vi "Flip Matrix.vi"(8 "Error In":errorcluster, 11 "Frame In":u32[][](array[numeric])) -> (0 "Error Out":errorcluster, 3 "Frame Out":u32[][](array[numeric]))   [LabVIEW 2019, in "Display.lvclass"]
uses:
  Display.lvclass
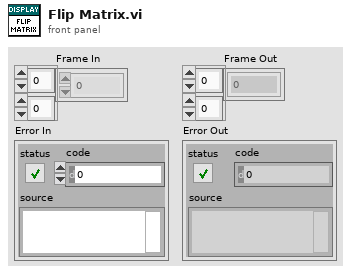
[diagram p1: front panel]
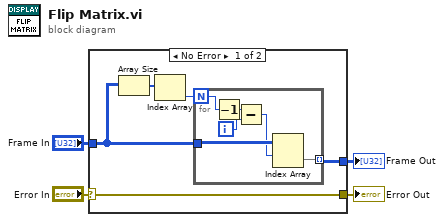
[diagram p0: block diagram]
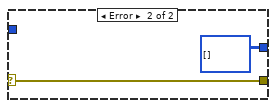
[diagram p2: hidden frame]
diagram:
  n1 = case shown="No Error" "Error In" {
    selector: "Error In" -> [w5 w17]
    tunnel: [w9 u32[][] [] ("Frame In")] -> w4
    tunnel: "Frame In" -> [w8 _]
    tunnel: [w5 w17] -> w1
    frame No Error {
      n2 = Array Size(array=w8) -> (size(s)=w6:i32[])
      n3 = Index Array(array=w6) -> (element=w7:i32)  [unwired: 1 in]
      n4 = for {
        N: w7 -> [w12]
        tunnel: w8 -> [w14]
        tunnel: [w10] -> w9 mode=indexing
        i -> [w15]
        n5 = Decrement(x=w12) -> (x-1=w11:i32)
        n6 = Subtract(x=w11, y=w15) -> (x-y=w13:i32)
        n7 = Index Array(array=w14, index (row)=w13) -> (element=w10:u32[])  [unwired: 1 in]
      }
    }
    frame Error {
    }
  }
  "Frame Out" <- w4
  "Error Out" <- w1
